vi "StatMon_AH2700.vi"(7 "System Monitor Variables":T1, 9 "Scale Meas Op":dbl=1.0, 11 "Update AH":bool) -> (0 "Meas Op Y":string, 1 "Meas Op X":string, 2 "Out 2":dbl[](array[numeric]), 3 "Out 1":dbl[](array[numeric]), 4 "Meas Op Z":string, 5 "Scaled":dbl[][](array[numeric]))   [LabVIEW 2016]
uses:
  Global/Global Variables/System Monitor Cluster.ctl
  Global/Global Variables/Data_Display_global.vi
panel:
  in  "Meas Op Ch 2":bool
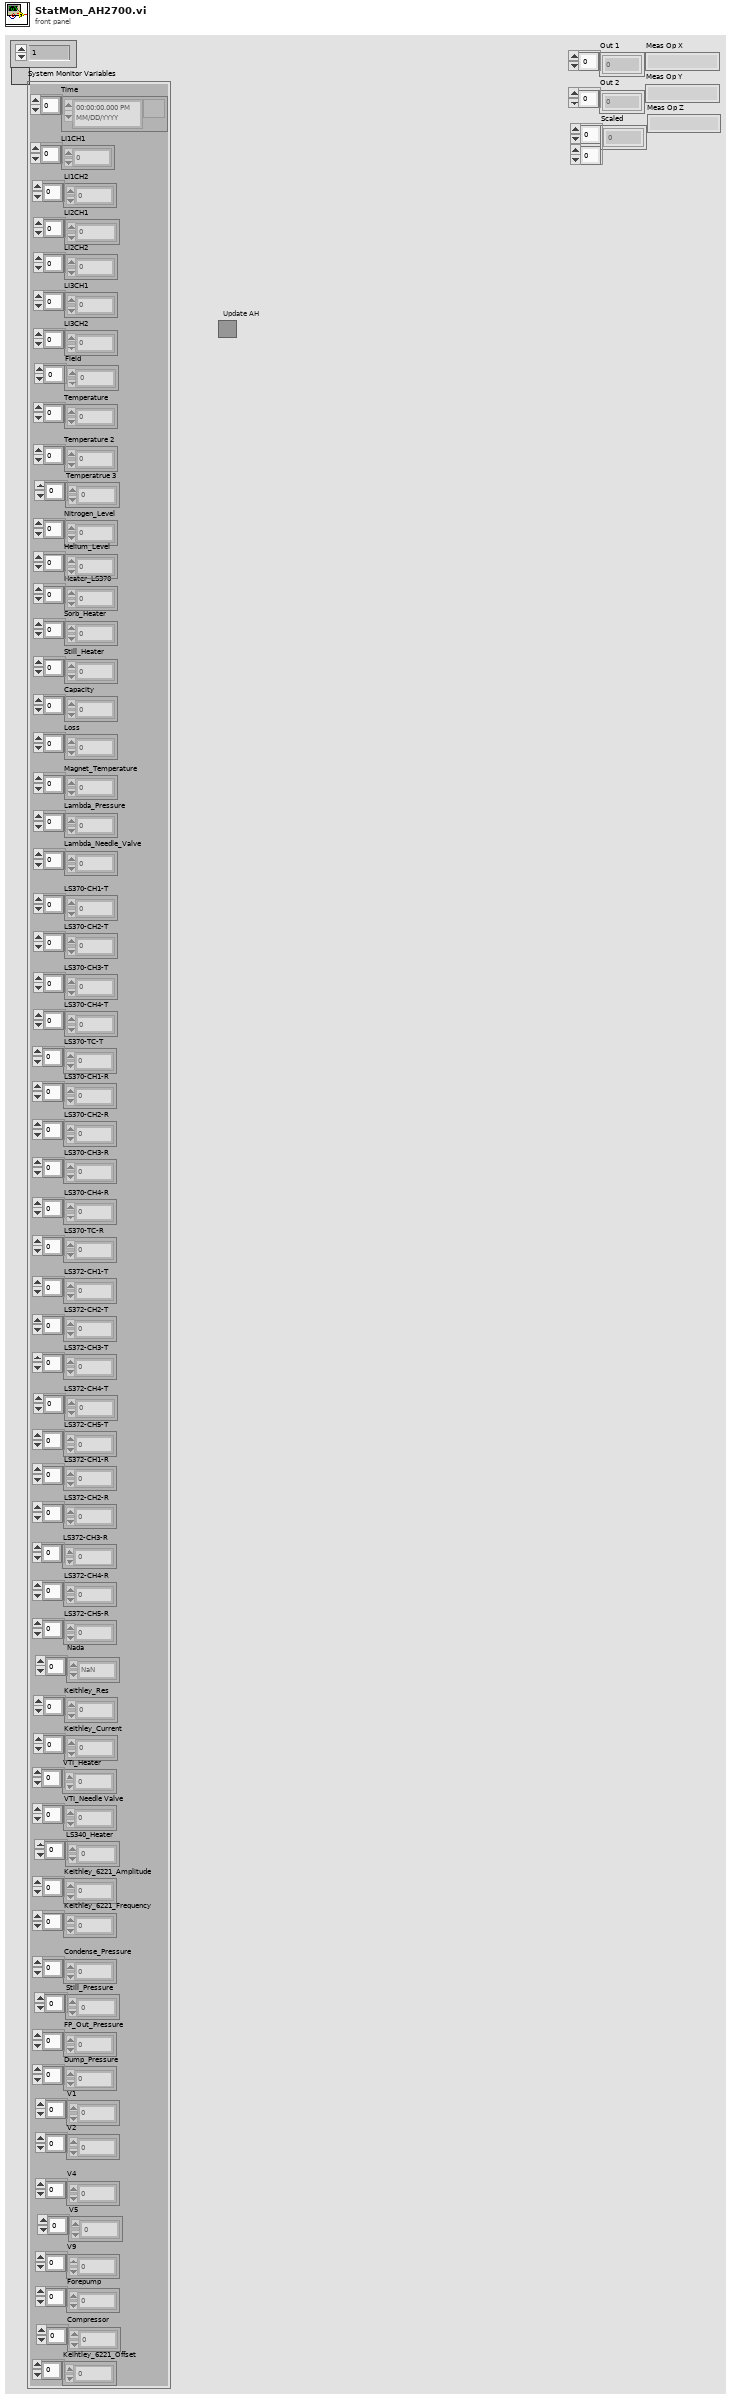
[diagram p1: front panel]
types:
  T1 = typedef "System Monitor Cluster.ctl" = cluster{"Time":timestamp[], "LI1CH1":dbl[], "LI1CH2":dbl[], "LI2CH1":dbl[], "LI2CH2":dbl[], "LI3CH1":dbl[], "LI3CH2":dbl[], "Field":dbl[], "Temperature":dbl[], "Temperature 2":dbl[], "Temperatrue 3":dbl[], "Nitrogen_Level":dbl[], "Helium_Level":dbl[], "Heater_LS370":dbl[], "Sorb_Heater":dbl[], "Still_Heater":dbl[], "Capacity":dbl[], "Loss":dbl[], "Magnet_Temperature":dbl[], "Lambda_Pressure":dbl[], "Lambda_Needle_Valve":dbl[], "LS370-CH1-T":dbl[], "LS370-CH2-T":dbl[], "LS370-CH3-T":dbl[], "LS370-CH4-T":dbl[], "LS370-TC-T":dbl[], "LS370-CH1-R":dbl[], "LS370-CH2-R":dbl[], "LS370-CH3-R":dbl[], "LS370-CH4-R":dbl[], "LS370-TC-R":dbl[], "LS372-CH1-T":dbl[], "LS372-CH2-T":dbl[], "LS372-CH3-T":dbl[], "LS372-CH4-T":dbl[], "LS372-CH5-T":dbl[], "LS372-CH1-R":dbl[], "LS372-CH2-R":dbl[], "LS372-CH3-R":dbl[], "LS372-CH4-R":dbl[], "LS372-CH5-R":dbl[], "Nada":dbl[], "Keithley_Res":dbl[], "Keithley_Current":dbl[], "VTI_Heater":dbl[], "VTI_Needle Valve":dbl[], "LS340_Heater":dbl[], "Keithley_6221_Amplitude":dbl[], "Keithley_6221_Frequency":dbl[], "Condense_Pressure":dbl[], "Still_Pressure":dbl[], "FP_Out_Pressure":dbl[], "Dump_Pressure":dbl[], "V1":dbl[], "V2":dbl[], "V4":dbl[], "V5":dbl[], "V9":dbl[], "Forepump":dbl[], "Compressor":dbl[], "Keihtley_6221_Offset":dbl[]}
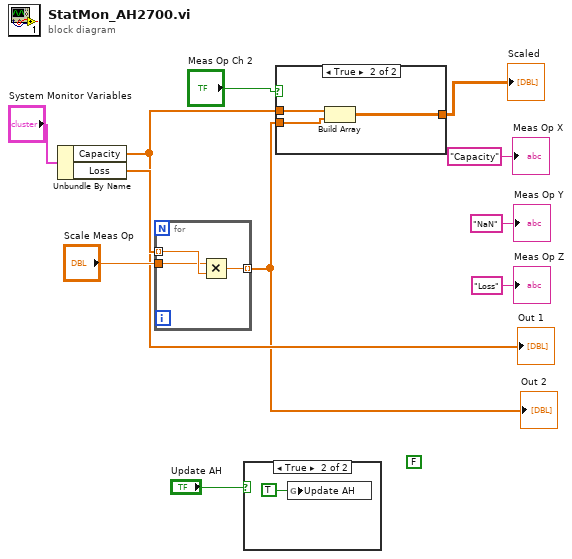
[diagram p0: block diagram]
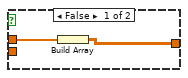
[diagram p2: hidden frame]
diagram:
  (unwired) FALSE
  n1 = Unbundle By Name("System Monitor Variables") -> ("Capacity"=w6:dbl[], "Loss"=w10:dbl[])
  "Out 1" <- w6
  n2 = for {
    tunnel: w10 -> [w14] mode=indexing
    tunnel: "Scale Meas Op" -> [w13]
    tunnel: [w12] -> w5 mode=indexing
    n3 = Multiply(x=w13, y=w14) -> (x*y=w12:dbl)
  }
  "Out 2" <- w5
  n4 = case shown="True" "Update AH" {
    frame False {
    }
    frame True {
      n5 = global write "Data_Display_global.vi" "Update AH"(TRUE) -> ()
    }
  }
  n6 = case shown="True" "Meas Op Ch 2" {
    tunnel: w6 -> [w17 w20]
    tunnel: [w16 w19] -> w1
    tunnel: w5 -> [_ w18]
    frame False {
      n7 = Build Array(w17) -> (w16:dbl[][])
    }
    frame True {
      n8 = Build Array(w20, w18) -> (w19:dbl[][])
    }
  }
  "Scaled" <- w1
  "Meas Op X" <- "Capacity"
  "Meas Op Y" <- "NaN"
  "Meas Op Z" <- "Loss"
